vi "calc_transform_matrix.vi"(10 "Translate":T1, 11 "Scale":T1) -> (3 "Transformation":sgl[][](array[numeric]))   [LabVIEW 2020, in "3DPC_SurfacePlot.xctl"]
uses:
  <vilib>/Native 3D Graph/xcontrol/3DPC_SurfacePlot.xctl
  <vilib>/Native 3D Graph/typedefs/vector.ctl
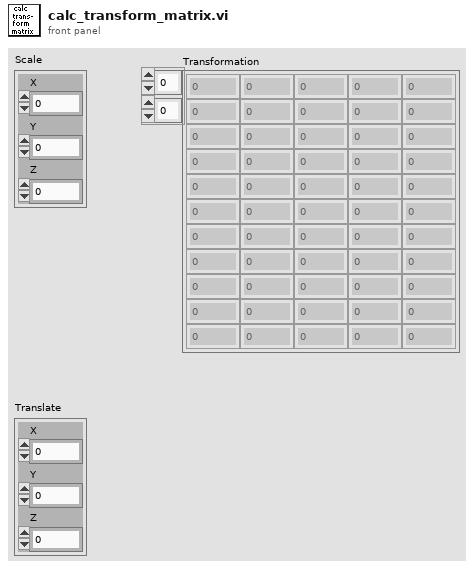
[diagram p1: front panel]
types:
  T1 = typedef "3DPC_SurfacePlot.xctl/vector.ctl" = cluster{"X":sgl, "Y":sgl, "Z":sgl}
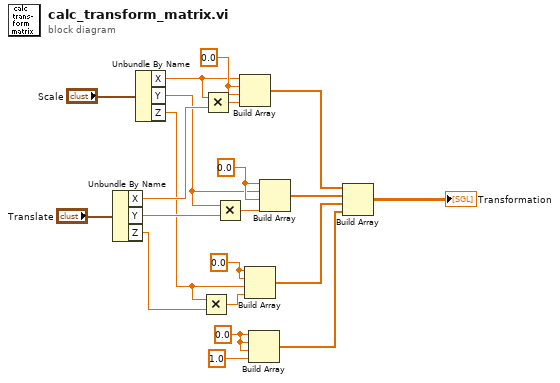
[diagram p0: block diagram]
diagram:
  w7 = 0.0 ("element")
  w11 = sgl 0.0 ("element")
  w15 = sgl 0.0 ("element")
  w19 = sgl 0.0 ("element")
  n1 = Unbundle By Name("Translate") -> ("X"=w16:sgl, "Y"=w13:sgl, "Z"=w8:sgl)
  n2 = Unbundle By Name("Scale") -> ("X"=w17:sgl, "Y"=w12:sgl, "Z"=w9:sgl)
  n3 = Multiply(x=w9, y=w8) -> (x*y=w10:sgl)
  n4 = Multiply(x=w17, y=w16) -> (x*y=w18:sgl)
  n5 = Multiply(x=w12, y=w13) -> (x*y=w14:sgl)
  n6 = Build Array(w17, w19, w19, w18) -> (w5:sgl[])
  n7 = Build Array(w11, w11, w9, w10) -> (w3:sgl[])
  n8 = Build Array(w7, w7, w7, 1.0 ("element")) -> (w2:dbl[])
  n9 = Build Array(w15, w12, w15, w14) -> (w4:sgl[])
  n10 = Build Array(w5, w4, w3, w2) -> (→"Transformation":dbl[][])
